vi "Write Data file path indicator ref.vi"(8 "error in (no error)":errorcluster, 10 "Data file path indicator ref":refnum<vi>, 11 "Spectrum Recorder in":refnum<class "Spectrum Recorder.lvclass">) -> (0 "error out":errorcluster, 3 "Spectrum Recorder out":refnum<class "Spectrum Recorder.lvclass">)   [LabVIEW 2016, in "Spectrum Recorder.lvclass"]
uses:
  Spectrum Recorder.lvclass
  Spectrum Recorder.lvclass/Spectrum Recorder.ctl
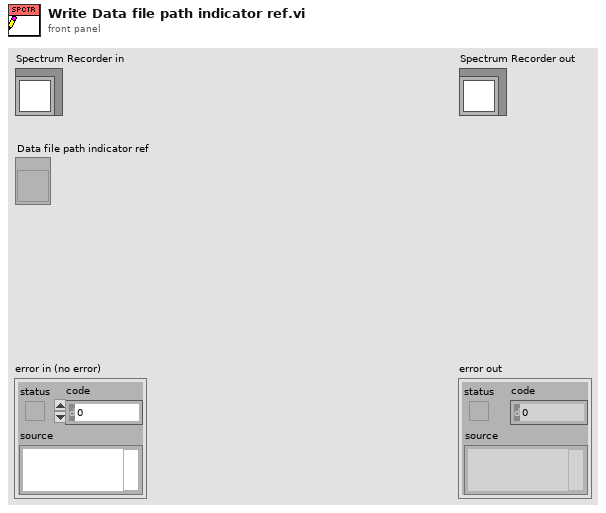
[diagram p1: front panel]
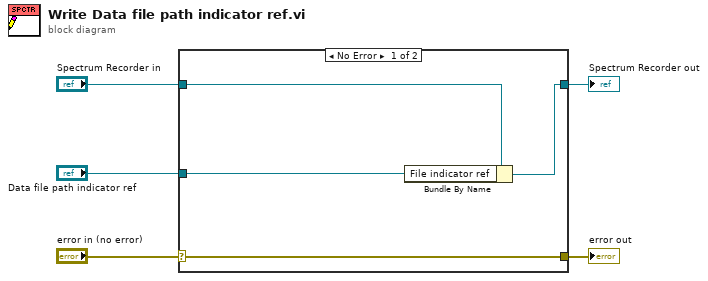
[diagram p0: block diagram]
diagram:
  n1 = case shown="No Error" "error in (no error)" {
    selector: "error in (no error)" -> [w9 w10]
    tunnel: [w9 w10] -> w4
    tunnel: [w7 w11] -> w2
    tunnel: "Spectrum Recorder in" -> [w8 w11]
    tunnel: "Data file path indicator ref" -> [w6 _]
    frame No Error {
      n2 = Bundle By Name(cluster=w8, "File indicator ref"=w6) -> (w7:refnum<class "Spectrum Recorder.lvclass">)
    }
    frame Error {
    }
  }
  "error out" <- w4
  "Spectrum Recorder out" <- w2
